vi "Close connection.vi"(8 "error in":errorcluster, 10 "abort (F)":bool, 11 "Connection Info":T1) -> (0 "error out":errorcluster, 3 "Connection Info out":T1)   [LabVIEW 2021]
uses:
  Connection Info.ctl
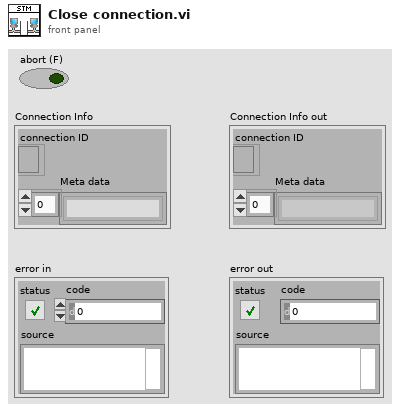
[diagram p1: front panel]
types:
  T1 = typedef "Connection Info.ctl" = cluster{"connection ID":refnum<k5>, "Meta data":string[]}
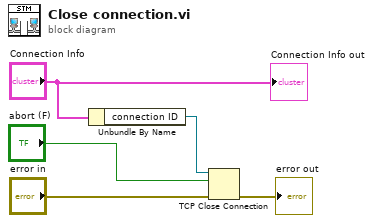
[diagram p0: block diagram]
diagram:
  n1 = Unbundle By Name("Connection Info") -> ("connection ID"=w5:refnum<k5>)
  n2 = TCP Close Connection(connection ID=w5, abort (F)="abort (F)", error in (no error)="error in") -> (error out=→"error out":errorcluster)  [unwired: 1 out]
  "Connection Info out" <- "Connection Info"
